vi "WriteToFifo.vi"(8 "error in (no error)":errorcluster, 9 "Timeout (ms)":i32=5000, 10 "Data":u32[](array[numeric]), 11 "FpgaInterface in":refnum<class "FpgaInterface.lvclass">) -> (0 "error out":errorcluster, 3 "FpgaInterface out":refnum<class "FpgaInterface.lvclass">)   [LabVIEW 2017, in "FpgaInterface.lvclass"]
uses:
  FpgaInterface.lvclass
  FpgaInterface.lvclass/FpgaInterface.ctl
  <vilib>/Utility/error.llb/Error Cluster From Error Code.vi
  <vilib>/rvi/errors/niLvFpgaAdjustHostInterfaceError.vi
  <vilib>/rvi/interface/nirviMethod/nirviMethod.xnode
  <vilib>/FPGAPlugInAG/Dynamic/niLvFpga_WriteFifo_Dynamic.vi
  <vilib>/rvi/errors/niLvFpgaMergeErrorWithErrorCode.vi
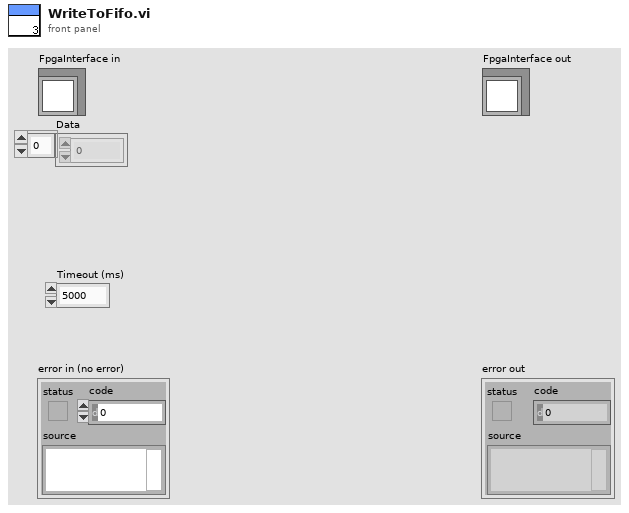
[diagram p1: front panel]
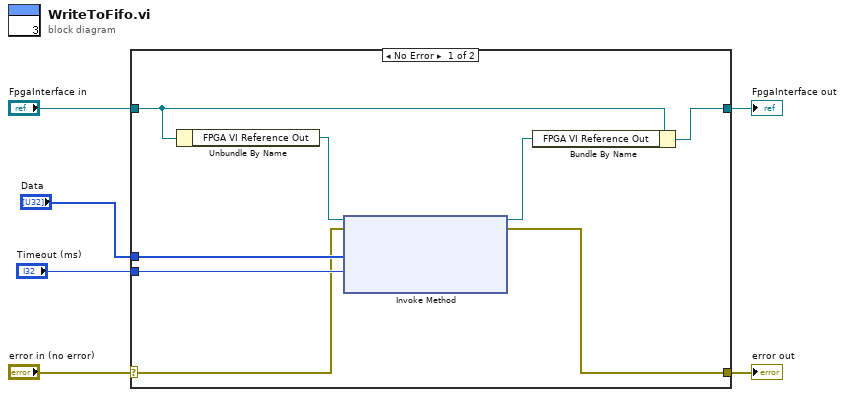
[diagram p0: block diagram]
diagram:
  n1 = case shown="No Error" "error in (no error)" {
    selector: "error in (no error)" -> [w11 w16]
    tunnel: [w10 w16] -> w5
    tunnel: [w7 w15] -> w3
    tunnel: "FpgaInterface in" -> [w8 w15]
    tunnel: "Timeout (ms)" -> [w13 _]
    tunnel: "Data" -> [w12 _]
    frame No Error {
      n2 = Unbundle By Name(w8) -> ("FPGA VI Reference Out"=w14:refnum<k20>)
      n3 = xnode "Invoke Method"("FPGA VI Reference In"=w14, "error in"=w11, "Data"=w12, "Timeout (ms)"=w13) -> ("FPGA VI Reference Out"=w9:refnum<k20>, "error out"=w10:errorcluster)  [unwired: 1 out]
      n4 = Bundle By Name(cluster=w8, "FPGA VI Reference Out"=w9) -> (w7:refnum<class "FpgaInterface.lvclass">)
    }
    frame Error {
    }
  }
  "error out" <- w5
  "FpgaInterface out" <- w3
